vi "Test Base Namer With Extension No Label.vi"(11 "Test Case In":refnum<class "Namer Tests.lvclass">) -> (0 "error out":errorcluster, 3 "Test Case Out":refnum<class "Namer Tests.lvclass">)   [LabVIEW 2020, in "Namer Tests.lvclass"]
uses:
  Namer Tests.lvclass
  C:/Program Files/National Instruments/LabVIEW 2026/vi.lib/Astemes/LUnit/Test Case.lvclass
  Source/Approval Tests/Namer/Namer.lvclass
  Source/Approval Tests/Naming Data/Naming Data.lvclass
  Source/Approval Tests/Naming Data/Naming Data.lvclass/Naming Data.ctl
  <vilib>/Astemes/LUnit/Test Case.lvclass/Test Case.ctl
  4993e8ee-a06a-463a-9684-69129f64d5ce.vi
  0918fd5e-94dd-4373-87d7-b18d263a6ff8.vi
  Source/Approval Tests/Naming Data/Write Test VI Name.vi
  Source/Approval Tests/Naming Data/Write Extension.vi
  <vilib>/Astemes/LUnit/Core/LUnit Test Case/Private/Append Pass Result.vi
  <vilib>/Astemes/LUnit/Core/LUnit Test Case/Private/Append Fail Result.vi
  4993e8ee-a06a-463a-9684-69129f64d5ce.vi/9c5d11cd-9439-4240-a1ee-d9baace9c924.vi
  0918fd5e-94dd-4373-87d7-b18d263a6ff8.vi/9c5d11cd-9439-4240-a1ee-d9baace9c924.vi
  <vilib>/Astemes/LUnit/Core/LUnit Test Case/Private/Run In UI.vi
  <vilib>/Utility/error.llb/Clear Errors.vi
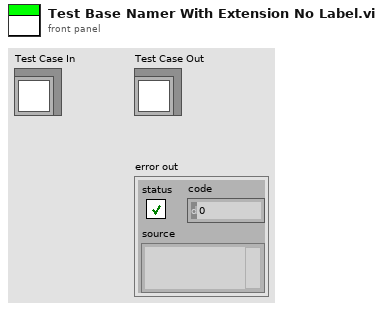
[diagram p1: front panel]
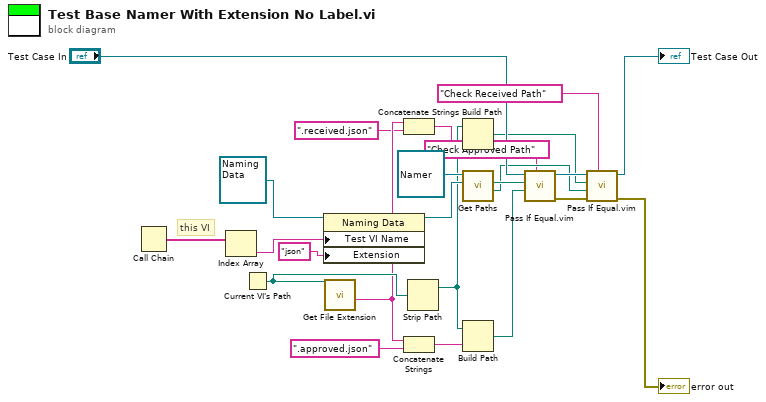
[diagram p0: block diagram]
diagram:
  # "this VI"
  n1 = Call Chain() -> (call chain=w19:string[])
  n2 = Index Array(array=w19) -> (element=w18:string)  [unwired: 1 in]
  n3 = Current VI's Path() -> (path=w16:path)
  n4 = property on="Property Node" class="Naming Data"(reference=refnum<class "Naming Data.lvclass"> refnum ("Naming Data"), "Test VI Name"=w18, "Extension"="json") -> (reference out=w17:refnum<class "Naming Data.lvclass">)  [unwired: 1 in, 1 out]
  n5 = call <vilib>:"Get File Extension.vi"("file"=w16) -> ("filename without extension"=w14:string)  [unwired: 6 in, 4 out]
  n6 = Concatenate Strings(w14, ".received.json" ("string")) -> (w11:string)
  n7 = Concatenate Strings(w14, ".approved.json" ("string")) -> (w10:string)
  n8 = Strip Path(path=w16) -> (stripped path=w15:path)  [unwired: 1 out]
  n9 = Build Path(base path=w15, name or relative path=w11) -> (appended path=w3:path)
  n10 = call-dynamic "Get Paths.vi"("Naming Data"=w17, "Namer in"=refnum<class "Namer.lvclass"> refnum ("Approval Tests:Namer")) -> ("Received Path"=w2:path, "Approved Path"=w8:path)  [unwired: 6 in, 2 out]
  n11 = Build Path(base path=w15, name or relative path=w10) -> (appended path=w7:path)
  n12 = call "Pass If Equal.vim"("Description"="Check Approved Path", "Actual"=w7, "Expected"=w8, "LUnit Test Case In"="Test Case In") -> ("error out"=w23:errorcluster, "LUnit Test Case Out"=w6:refnum<class "Namer Tests.lvclass">)  [unwired: 6 in]
  n13 = call "Pass If Equal.vim"("Description"="Check Received Path" ("Label (VI Title)"), "error in (no error)"=w23, "Actual"=w2, "Expected"=w3, "LUnit Test Case In"=w6) -> ("error out"=→"error out":errorcluster, "LUnit Test Case Out"=→"Test Case Out":refnum<class "Namer Tests.lvclass">)  [unwired: 5 in]
